vi "ResetBins.vi"(8 "error in":errorcluster, 10 "Reset?":bool, 11 "Channel Data in":i32[](array[numeric])) -> (0 "error out":errorcluster, 3 "Channel Data out":i32[](array[numeric]))   [LabVIEW 2012, in "Histogram Custom Device.lvlib"]
uses:
  Histogram Custom Device.lvlib
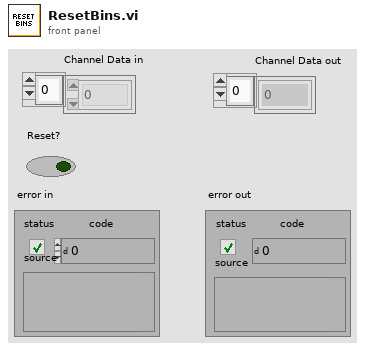
[diagram p1: front panel]
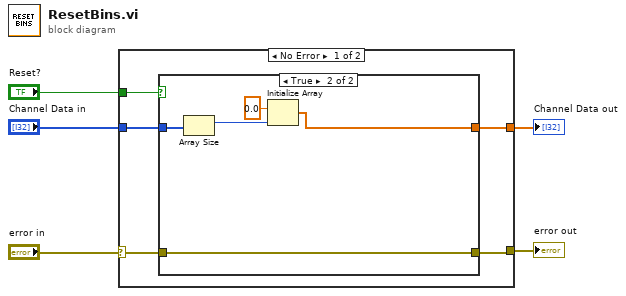
[diagram p0: block diagram]
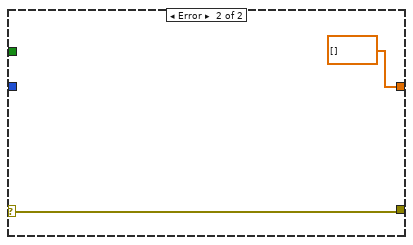
[diagram p3: hidden frame]
diagram:
  n1 = case shown="No Error" "error in" {
    selector: "error in" -> [w7 w19]
    tunnel: [w8 dbl[] []] -> w5
    tunnel: [w6 w19] -> w3
    tunnel: "Channel Data in" -> [w9 _]
    tunnel: "Reset?" -> [w10 _]
    frame No Error {
      n2 = case shown="True" w10 {
        tunnel: [w12 w14] -> w8
        tunnel: w9 -> [w12 w17]
        tunnel: w7 -> [w11 w13]
        tunnel: [w11 w13] -> w6
        frame False {
        }
        frame True {
          n3 = Array Size(array=w17) -> (size(s)=w16:i32)
          n4 = Initialize Array(0.0 ("element"), w16) -> (w14:dbl[])
        }
      }
    }
    frame Error {
    }
  }
  "Channel Data out" <- w5
  "error out" <- w3
